vi "Global.vi"() -> ()   [LabVIEW 2017]
uses:
  LT_UpgradeFlash.lvclass
panel:
  out "LT_Class_ref":refnum<class "LT_UpgradeFlash.lvclass">
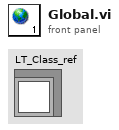
[diagram p1: front panel]
diagram:
